vi "append lines to loggfile (sub-vi).vi"(8 "error in (no error)":errorcluster, 10 "string array":string[](array[string]), 11 "file refnum":refnum<file>) -> (0 "error out":errorcluster, 3 "file refnum out":refnum<file>)   [LabVIEW 2021]
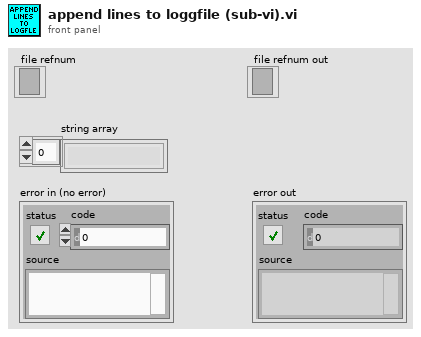
[diagram p1: front panel]
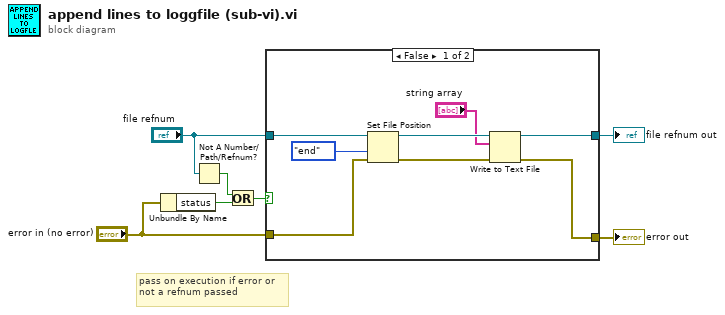
[diagram p0: block diagram]
diagram:
  # "pass on execution if error or \nnot a refnum passed"
  n1 = Unbundle By Name("error in (no error)") -> ("status"=w1:bool)
  n2 = Not A Number/Path/Refnum?(number/path/refnum="file refnum") -> (NaN/Path/Refnum?=w4:bool)
  n3 = Or(x=w4, y=w1) -> (x .or. y?=w3:bool)
  n4 = case shown="False" w3 {
    tunnel: [w15 w17] -> w7
    tunnel: [w10 w16] -> w6
    tunnel: "file refnum" -> [w9 w17]
    tunnel: "error in (no error)" -> [w8 w16]
    frame False {
      n5 = Set File Position(refnum=w9, from (0:start)=enum16{"start", "end", "current"}."end", error in=w8) -> (refnum out=w14:refnum<file>, error out=w13:errorcluster)  [unwired: 1 in]
      n6 = Write to Text File(file (use dialog)=w14, text="string array", error in=w13) -> (refnum out=w15:refnum<file>, error out=w10:errorcluster)  [unwired: 1 in, 1 out]
    }
    frame True {
    }
  }
  "file refnum out" <- w7
  "error out" <- w6
